vi "Load Scan.vi"(8 "error in (no error)":errorcluster, 11 "XML File Path":path) -> (0 "error out":errorcluster, 3 "Scan Driver out":refnum<class "Scan Driver.lvclass">)   [LabVIEW 2009, in "Scan Driver.lvclass"]
doc: "Unflattens a Scan Driver instance from the specified XML file. If an error occurs, returns the class default object."
uses:
  Scan Driver.lvclass
  <vilib>/Utility/xml.llb/Read From XML File(string).vi
  Scan Driver.lvclass/Scan Driver.ctl
  Scanners/Scanner/Scanner.lvclass
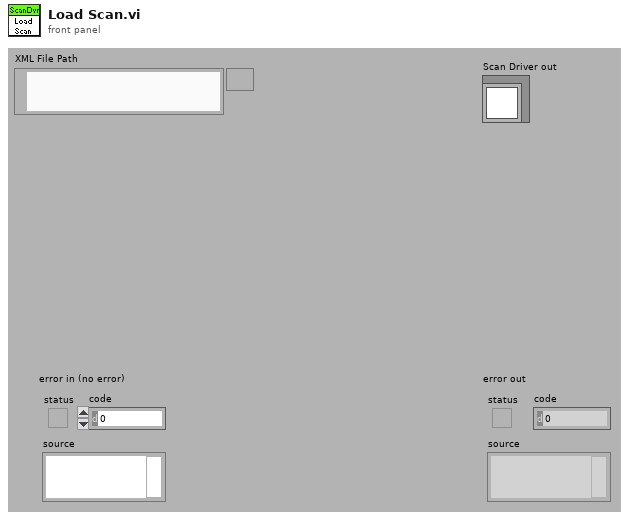
[diagram p1: front panel]
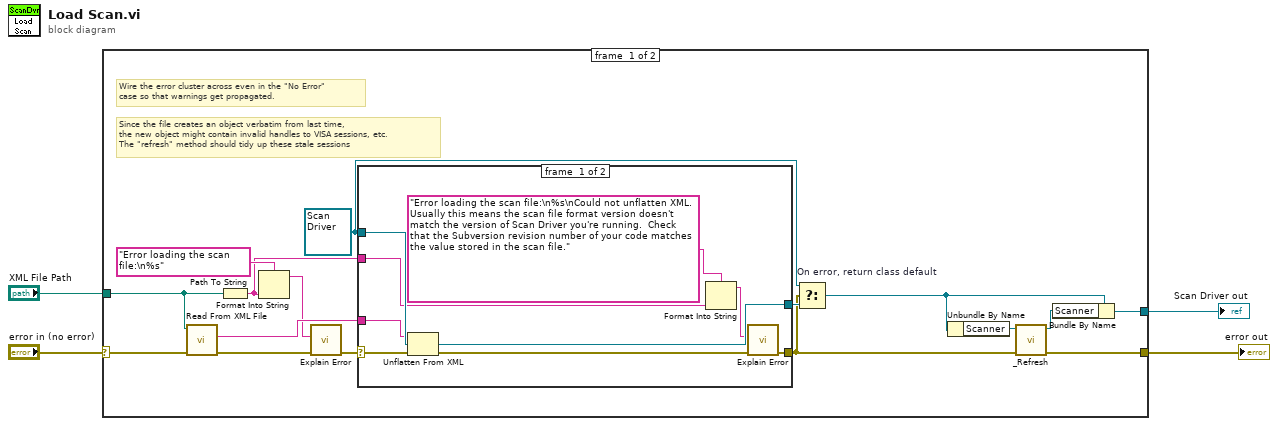
[diagram p0: block diagram]
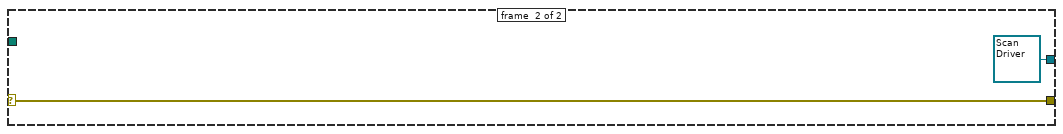
[diagram p3: hidden frame]
diagram:
  n1 = case shown="No Error" "error in (no error)" {
    selector: "error in (no error)" -> [w12 w33]
    tunnel: [w5 w33] -> w3
    tunnel: [w10 refnum<class "Scan Driver.lvclass"> refnum ("Scan Driver out")] -> w2
    tunnel: "XML File Path" -> [w17 _]
    frame #0 {
      w19 = refnum<class "Scan Driver.lvclass"> refnum ("Scan Driver out")
      # "Since the file creates an object verbatim from last time,\nthe new object might contain invalid handles to VISA sessions, etc.\nThe \"refresh\" method should tidy up these stale sessions"
      # "Wire the error cluster across even in the \"No Error\"\ncase so that warnings get propagated."
      n2 = call-poly <vilib>:"Read From XML File.vi"("error in (no error)"=w12, "XML File Path"=w17) -> ("error out"=w8:errorcluster, "XML Elements"=w18:string)  [unwired: 8 out]
      n3 = Path To String(path=w17) -> (string=w15:string)
      n4 = Format Into String(format string="Error loading the scan file:\n%s" ("error message (\"\")"), w15) -> (resulting string=w6:string)  [unwired: 2 in, 1 out]
      n5 = call "Explain Error.vi"("error in"=w8, "Explanation"=w6) -> ("error out"=w7:errorcluster)  [unwired: 9 out]
      n6 = case shown="No Error" w7 {
        selector: w7 -> [w26 w31]
        tunnel: [w29 w30] -> w20
        tunnel: w19 -> [w28 w30]
        tunnel: w18 -> [w27 _]
        tunnel: [w21 w31] -> w9
        tunnel: w15 -> [w24 _]
        frame #0 {
          n7 = Unflatten From XML(xml string=w27, type=w28, error in (no error)=w26) -> (value=w29:refnum<class "Scan Driver.lvclass">, error out=w22:errorcluster)
          n8 = Format Into String(format string="Error loading the scan file:\n%s\nCould not unflatten XML.  Usually this means the scan file format version doesn't match the version of Scan Driver you're running.  Check that the Subversion revision number of your code matches the value stored in the scan file.", w24) -> (resulting string=w23:string)  [unwired: 2 in, 1 out]
          n9 = call "Explain Error.vi"("error in"=w22, "Explanation"=w23) -> ("error out"=w21:errorcluster)  [unwired: 9 out]
        }
        frame #1 {
        }
      }
      n10 = Select "On error, return class default"(t=w19, s=w9, f=w20) -> (s? t:f=w11:refnum<class "Scan Driver.lvclass">)
      n11 = Unbundle By Name(w11) -> ("Scanner"=w14:refnum<class "Scanner.lvclass">)
      n12 = call-dynamic "_Refresh.vi"("error in (no error)"=w9, "Scanner in"=w14) -> ("error out"=w5:errorcluster, "Scanner out"=w13:refnum<class "Scanner.lvclass">)  [unwired: 8 out]
      n13 = Bundle By Name(cluster=w11, "Scanner"=w13) -> (w10:refnum<class "Scan Driver.lvclass">)
    }
    frame #1 {
    }
  }
  "error out" <- w3
  "Scan Driver out" <- w2
